vi "Get MicronGRPC Message Request.vi"(8 "error in (no error)":errorcluster, 11 "gRPCid":T1) -> (0 "error out":errorcluster, 2 "Message Data":T2, 3 "gRPCid out":T1)   [LabVIEW 2019, in "MicronGRPCGeneratedServer.lvlib" / "MicronGRPC.lvclass"]
uses:
  MicronGRPC.lvclass
  RPC Messages/micronGrpc_MessageRequest.ctl
  <vilib>/gRPC/LabVIEW gRPC Library/Shared/grpcId.ctl
  MicronGRPCGeneratedServer.lvlib
  <vilib>/gRPC/LabVIEW gRPC Library/grpc-lvsupport-release.lvlib
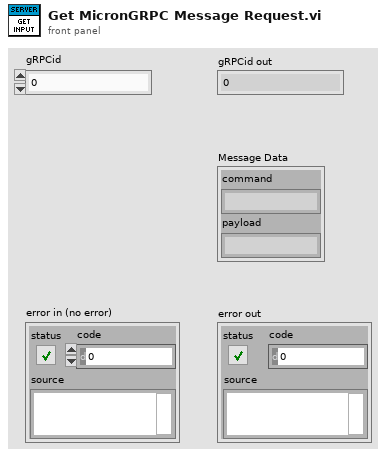
[diagram p1: front panel]
types:
  T1 = typedef "grpc-lvsupport-release.lvlib/grpcId.ctl" = u64
  T2 = typedef "MicronGRPCGeneratedServer.lvlib/micronGrpc_MessageRequest.ctl" = cluster{"command":string, "payload":string}
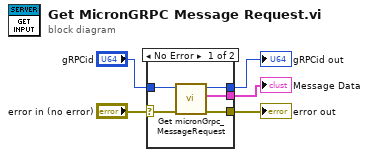
[diagram p0: block diagram]
diagram:
  n1 = case shown="No Error" "error in (no error)" {
    selector: "error in (no error)" -> [w10 w12]
    tunnel: [w9 w12] -> w4
    tunnel: [w8 _] -> w3
    tunnel: "gRPCid" -> [w7 w11]
    tunnel: [w6 w11] -> w1
    frame No Error {
      n2 = call "Get micronGrpc_MessageRequest.vi"("error in (no error)"=w10, "gRPCid"=w7) -> ("error out"=w9:errorcluster, "package_templatemessage"=w8:T2, "gRPCid out"=w6:T1)  [unwired: 7 in]
    }
    frame Error {
    }
  }
  "error out" <- w4
  "Message Data" <- w3
  "gRPCid out" <- w1
